vi "Configure Markers.vi"(4 "Stop Address (1)":dbl=1.0, 6 "Start Address (0)":dbl, 7 "Marker Pattern":bool[](array[boolean]), 8 "error in (no error)":errorcluster, 9 "Set Marker (0: Single Marker)":u16(ring) items=["Single Marker", "Marker Pattern"], 10 "Arbitrary Waveform Name":string, 11 "VISA resource name":refnum<visa-resource-name>) -> (0 "error out":errorcluster, 3 "VISA resource name out":refnum<visa-resource-name>)   [LabVIEW 2015, in "Fluke 28x Series.lvlib"]
doc: "Sets single or multiple markers in an already existing arbitrary waveform. \n\n<b>Note</b>: This VI only applies to arbitrary waveforms."
uses:
  <instrlib>/Fluke 28x Series/Fluke 28x Series.lvlib
panel:
  # "Set Marker Pattern"
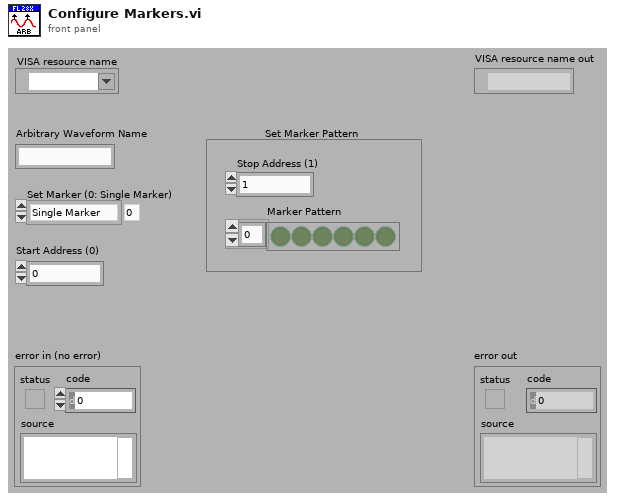
[diagram p1: front panel]
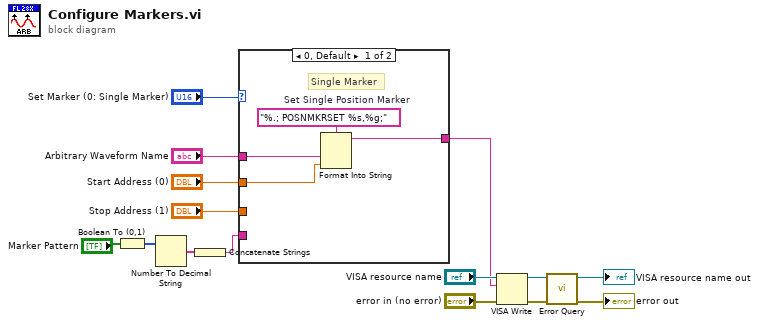
[diagram p0: block diagram]
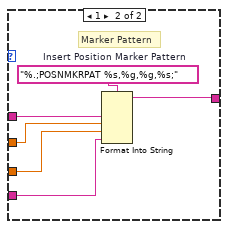
[diagram p2: hidden frame]
diagram:
  n1 = Boolean To (0,1)(Boolean="Marker Pattern") -> (0, 1=w6:i16[])
  n2 = Number To Decimal String(number=w6) -> (decimal integer string=w5:string[])  [unwired: 1 in]
  n3 = Concatenate Strings(w5) -> (w4:string)
  n4 = case shown="0, Default" "Set Marker (0: Single Marker)" {
    tunnel: "Arbitrary Waveform Name" -> [w18 w23]
    tunnel: "Start Address (0)" -> [w17 w22]
    tunnel: [w16 w24] -> w7
    tunnel: "Stop Address (1)" -> [_ w21]
    tunnel: w4 -> [_ w20]
    frame 0, Default {
      w19 = "%.; POSNMKRSET %s,%g;"  # Set Single Position Marker
      # "Single Marker"
      n5 = Format Into String(format string=w19, w18, w17) -> (resulting string=w16:string)  [unwired: 2 in, 1 out]
    }
    frame 1 {
      w25 = "%.;POSNMKRPAT %s,%g,%g,%s;"  # Insert Position Marker Pattern
      # "Marker Pattern"
      n6 = Format Into String(format string=w25, w23, w22, w21, w20) -> (resulting string=w24:string)  [unwired: 2 in, 1 out]
    }
  }
  n7 = VISA Write(VISA resource name="VISA resource name", write buffer=w7, error in (no error)="error in (no error)") -> (VISA resource name out=w11:refnum<visa-resource-name>, error out=w10:errorcluster)  [unwired: 1 out]
  n8 = call <instrlib>:"Error Query.vi"("error in (no error)"=w10, "VISA resource name"=w11) -> ("error out"=→"error out":errorcluster, "VISA resource name out"=→"VISA resource name out":refnum<visa-resource-name>)  [unwired: 6 in, 2 out]
